vi "DMM_Measure.vi"(0 "Semiconductor Module Context":T1, 5 "Pins":string[](array[string])=["RF1"], 11 "Error In":errorcluster) -> (4 "Semiconductor Module Context Out":T1, 6 "Measurement":dbl[](array[numeric]), 15 "Error Out":errorcluster)   [LabVIEW 2013]
uses:
  <vilib>/NI_TestStand_SemiconductorModule/NI_TestStand_Semiconductor_Module.lvlibp/PinMap/General/SemiconductorModuleContext.ctl
  Pin Map API/DMM Custom Instruments.lvlib
  <vilib>/NI_TestStand_SemiconductorModule/NI_TestStand_Semiconductor_Module.lvlibp
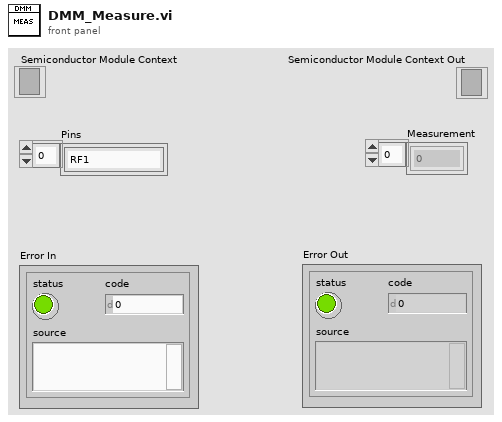
[diagram p1: front panel]
types:
  T1 = typedef "NI_TestStand_Semiconductor_Module.lvlibp/SemiconductorModuleContext.ctl" = refnum<k7>
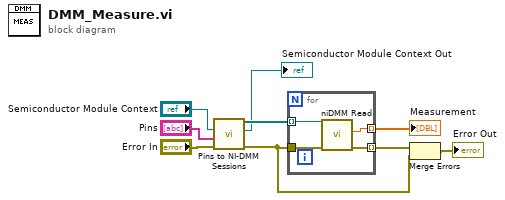
[diagram p0: block diagram]
diagram:
  n1 = call "Pins to NI-DMM Sessions.vi"("error in (no error)"="Error In", "Pins"="Pins", "Semiconductor Module Context"="Semiconductor Module Context") -> ("error out"=w5:errorcluster, "Semiconductor Module Context Out"=→"Semiconductor Module Context Out":T1, "Instrument Sessions"=w6:refnum<k15>[])  [unwired: 4 in, 2 out]
  n2 = for {
    tunnel: w6 -> [w13] mode=indexing
    tunnel: w5 -> [w12]
    tunnel: [w10] -> w2 mode=indexing
    tunnel: [w11] -> w1 mode=indexing
    n3 = call <instrlib>:"niDMM Read.vi"("error in (no error)"=w12, "instrument handle"=w13) -> ("error out"=w10:errorcluster, "Measurement"=w11:dbl)  [unwired: 7 in, 1 out]
  }
  "Measurement" <- w1
  n4 = Merge Errors(w2, w5) -> (→"Error Out":errorcluster)
